vi "A1343 CRC (1).vi"(0 "Data":u8[](array[numeric])=[12, 5, 0] format="%x") -> (4 "CRC":u8 format="%x")   [LabVIEW 2013]
doc: "This VI calculates the checksum required for outgoing and incoming SENT data."
panel:
  # "CRC-4"
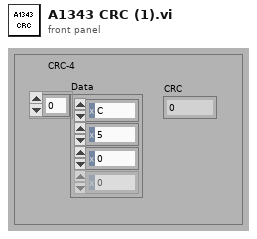
[diagram p1: front panel]
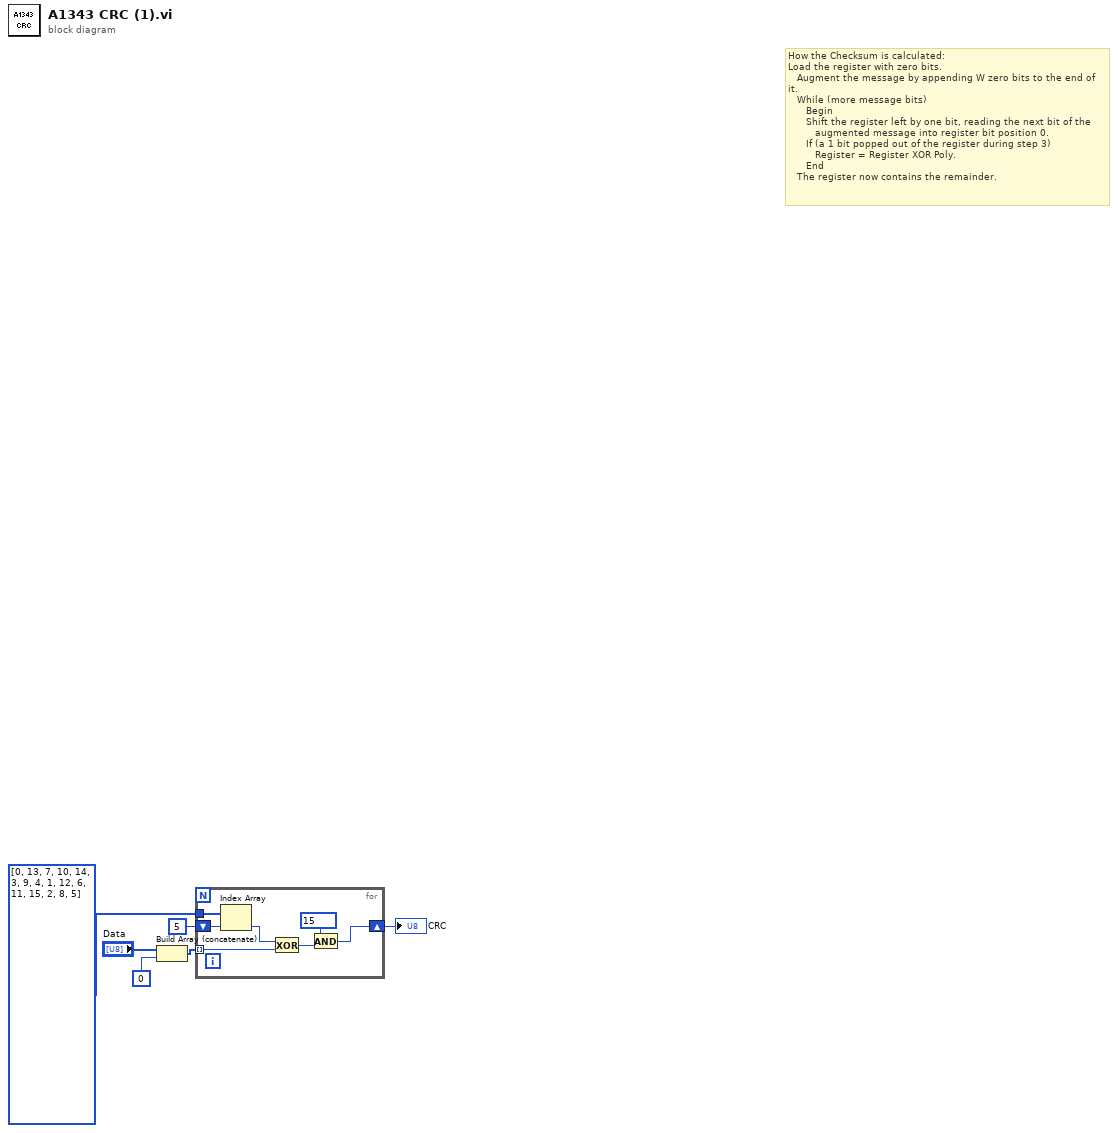
[diagram p0: block diagram]
diagram:
  # "How the Checksum is calculated:\nLoad the register with zero bits.\n   Augment the message by appending W zero bits to the end of it.\n   While (more message bits)\n      Begin\n      Shift the register left by one bit, reading the next bit of the\n         augmented message into register bit position 0.\n      If (a 1 bit popped out of the register during step 3)\n         Register = Register XOR Poly.\n      End\n   The register now contains the remainder."
  n1 = Build Array (concatenate)("Data", u8 0) -> (w2:u8[])
  n2 = for {
    tunnel: w2 -> [w12] mode=indexing
    shift-right: [w8] -> w4
    shift-left: u8 5 ("x") -> [w7]
    tunnel: u8[] [0, 13, 7, 10, 14, 3, 9, 4, 1, 12, 6, 11, 15, 2, 8, 5] ("Data 4") -> [w13]
    n3 = Index Array(array=w13, index=w7) -> (element=w11:u8)
    n4 = Exclusive Or(1:w12, 2:w11) -> (0:w9:u8)
    n5 = And(x=u8 15, y=w9) -> (x .and. y?=w8:u8)
  }
  "CRC" <- w4
